vi "receive twitter command.vi"(8 "error in":errorcluster) -> (0 "error out":errorcluster, 2 "New Tweets Read":T5[](array[typedef]), 3 "Time Stamp of Oldest Tweet":timestamp)   [LabVIEW 2019]
uses:
  <vilib>/LVH/i3 Twitter/Controls/Tweet.ctl
  <vilib>/LVH/i3 Twitter/Controls/Twitter Handle.ctl
  <vilib>/LVH/i3 OAuth/Controls/OAuth Handle.ctl
  <vilib>/LVH/i3 OAuth/Controls/Signature Method.ctl
  <vilib>/LVH/i3 OAuth/Controls/Credentials.ctl
  <vilib>/LVH/i3 Twitter/SubVIs/Twitter Open - Embedded.vi
  <vilib>/LVH/i3 Twitter/Tweets/Get Tweets Old.vi
  <vilib>/LVH/i3 Twitter/i3-twitter.lvlib
  <vilib>/LVH/i3 OAuth/i3-oauth.lvlib
panel:
  out "Actual Num of Tweets Read":i32
  out "Twitter Handle Out":T1={"OAuth Credentials"={"Signature Method"=enum."HMAC-SHA1", "Version"="1.0", "Client"={"Token"="", "Secret"=""}, "Access"={"Token"="", "Secret"=""}}, "since ID"="", "max ID"="", "Screen Name"=""}
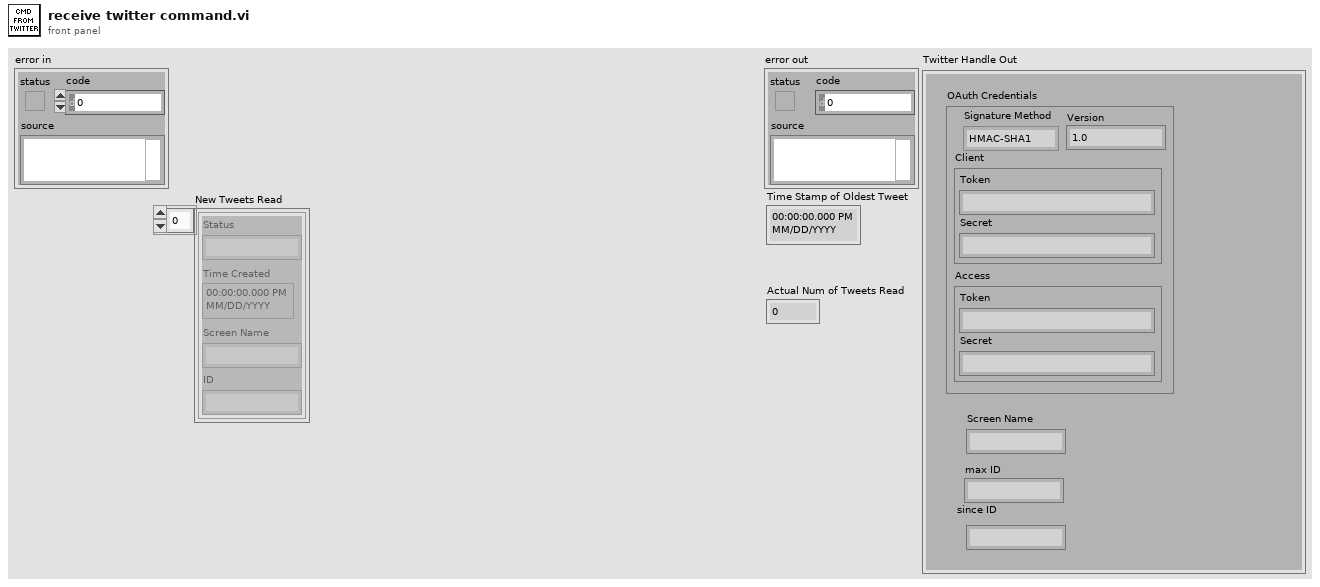
[diagram p1: front panel]
types:
  T1 = typedef "i3-twitter.lvlib/Twitter Handle.ctl" = cluster{"OAuth Credentials":T2, "since ID":string, "max ID":string, "Screen Name":string}
  T2 = typedef "i3-oauth.lvlib/OAuth Handle.ctl" = cluster{"Signature Method":T3, "Version":string, "Client":T4, "Access":T4}
  T3 = typedef "i3-oauth.lvlib/Signature Method.ctl" = enum16{"HMAC-MD5", "HMAC-SHA1", "HMAC-SHA224", "HMAC-SHA256", "HMAC-SHA384", "HMAC-SHA512"}
  T4 = typedef "i3-oauth.lvlib/Credentials.ctl" = cluster{"Token":string, "Secret":string}
  T5 = typedef "i3-twitter.lvlib/Tweet.ctl" = cluster{"Status":string, "Time Created":timestamp, "Screen Name":string, "ID":string}
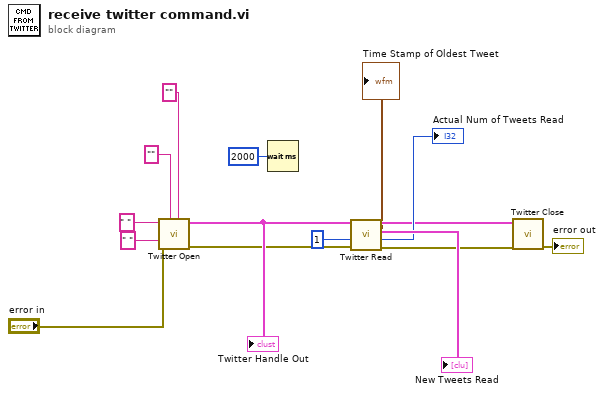
[diagram p0: block diagram]
diagram:
  n1 = call-poly <vilib>:"Twitter Open.vi"("Access Secret"="", "Access Token"="", "error in"="error in", "Consumer Secret"=" ", "Consumer Key"=" ") -> ("error out"=w14:errorcluster, "Twitter Handle Out"=w15:T1)  [unwired: 5 in]
  "Twitter Handle Out" <- w15
  n2 = Wait (ms)(milliseconds to wait=u32 2000) -> ()  [unwired: 1 out]
  n3 = call-poly <vilib>:"Twitter Read.vi"("error in"=w14, "Tweets to Read (10)"=1, "Twitter Handle In"=w15) -> ("error out"=w6:errorcluster, "Actual Num of Tweets Read"=→"Actual Num of Tweets Read":i32, "Old Tweets Read"=→"New Tweets Read":T5[], "Twitter Handle Out"=w4:T1, "Time Stamp of Oldest Tweet"=→"Time Stamp of Oldest Tweet":timestamp)  [unwired: 4 in]
  n4 = call <vilib>:"Twitter Close.vi"("error in"=w6, "Twitter Handle In"=w4) -> ("error out"=→"error out":errorcluster)  [unwired: 9 in]
